vi "FTW-SQLite-ExecuteScript.vi"(0 "SQLite Connector":refnum<class "FTW-SQLite-Connector.lvclass">, 5 "SQL Script":string, 11 "error in":errorcluster) -> (4 "SQLite Connector out":refnum<class "FTW-SQLite-Connector.lvclass">, 6 "Time to Execute+Compile":dbl format="%.6fsec", 8 "Time to Compile SQL":dbl format="%.6fsec", 15 "error out":errorcluster)   [LabVIEW 2013, in "FTW-SQLite-Connector.lvclass"]
uses:
  FTW-SQLite-Connector.lvclass
panel:
  # "Inputs"
  # "Outputs"
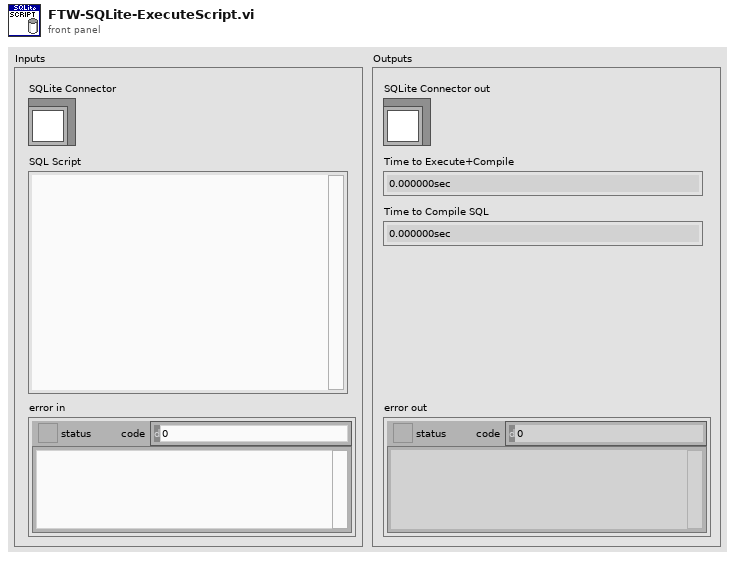
[diagram p1: front panel]
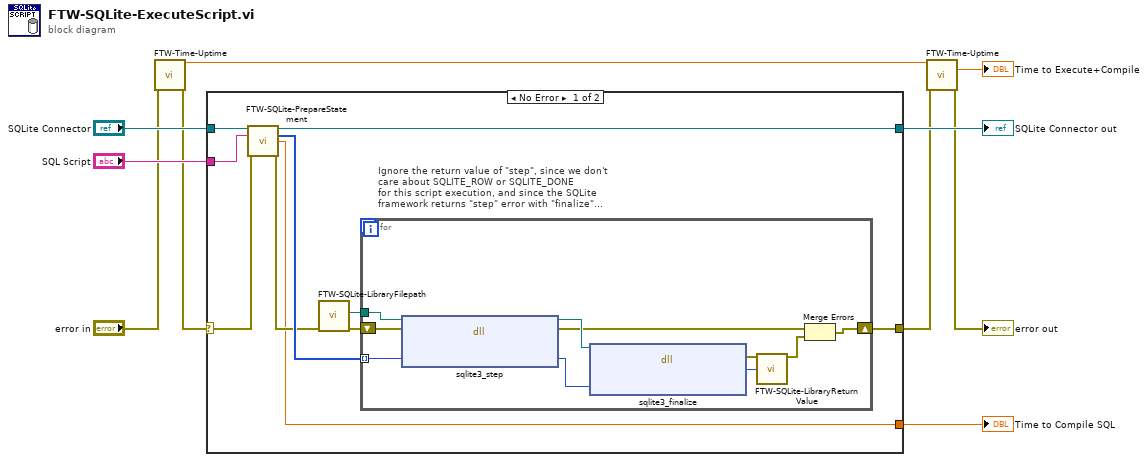
[diagram p0: block diagram]
diagram:
  n1 = call "FTW-Time-Uptime.vi"("error in"="error in") -> ("Current Uptime"=w5:dbl, "error out"=w6:errorcluster)  [unwired: 12 in, 1 out]
  n2 = case shown="No Error" w6 {
    selector: w6 -> [w19 w31]
    tunnel: "SQLite Connector" -> [w20 w32]
    tunnel: [w18 w32] -> w9
    tunnel: "SQL Script" -> [w17 _]
    tunnel: [w12 w31] -> w3
    tunnel: [w11 _] -> w1
    frame No Error {
      n3 = call "FTW-SQLite-PrepareStatement.vi"("SQLite Connector"=w20, "SQL Statement"=w17, "error in"=w19) -> ("SQLite Connector out"=w18:refnum<class "FTW-SQLite-Connector.lvclass">, "Prepared Statements"=w16:i64[], "Time to Compile SQL"=w11:dbl, "error out"=w15:errorcluster)  [unwired: 9 in]
      n4 = call "FTW-SQLite-LibraryFilepath.vi"("error in"=w15) -> ("error out"=w14:errorcluster, "SQLite Library Filepath"=w13:path)  [unwired: 8 in, 1 out]
      n5 = for "Ignore the return value of \"step\", since we don't care about SQLITE_ROW or SQLITE_DONE\nfor this script execution, and since the SQLite framework returns \"step\" error with \"finalize\"\nanyway. Also, we \"finalize\" every prepared statement unconditionally of upstream errors,\nbut only execute \"step\" if no upstream errors." {
        tunnel: w16 -> [w28] mode=indexing
        shift-right: [w22] -> w12
        shift-left: w14 -> [w30]
        tunnel: w13 -> [w29]
        n6 = dll-call lib="?" fn="sqlite3_step"(path in=w29, error in=w30, "Prepared Statement Pointer"=w28) -> (path out=w24:path, error out=w23:errorcluster, "Prepared Statement Pointer"=w27:i64)  [unwired: 2 in]
        n7 = dll-call lib="?" fn="sqlite3_finalize"(path in=w24, "Prepared Statement Pointer"=w27) -> (error out=w26:errorcluster, "Return Value"=w25:i32)  [unwired: 3 in, 1 out]
        n8 = call "FTW-SQLite-LibraryReturnValue.vi"("error in"=w26, "Return Value"=w25) -> ("error out"=w21:errorcluster)  [unwired: 13 in]
        n9 = Merge Errors(w23, w21) -> (w22:errorcluster)
      }
    }
    frame Error {
    }
  }
  "SQLite Connector out" <- w9
  "Time to Compile SQL" <- w1
  n10 = call "FTW-Time-Uptime.vi"("Previous Uptime"=w5, "error in"=w3) -> ("Elapsed Time"=→"Time to Execute+Compile":dbl, "error out"=→"error out":errorcluster)  [unwired: 11 in, 1 out]
